vi "11-async.vi"() -> ()   [LabVIEW 2018, in "LV2Julia_examples.lvlib"]
uses:
  LV2Julia_examples.lvlib
  LV2Julia_core/VIs/Server or client state.ctl
  LV2Julia_core/VIs/detailed error info.ctl
  LV2Julia_core/VIs/StackFrame.ctl
  LV2Julia_core/VIs/Commands.ctl
  be4745b6-8471-45fc-b8a0-8968ce92ea4b.vi
  877f6708-f4bd-42a3-8abe-32eb8c2c970e.vi
  be4745b6-8471-45fc-b8a0-8968ce92ea4b.vi/01ce1741-ea78-47f8-98ed-e79163fb1a9b.vi
  877f6708-f4bd-42a3-8abe-32eb8c2c970e.vi/896d20f1-cb1d-4420-8f1f-f93355f5adea.vi
  be4745b6-8471-45fc-b8a0-8968ce92ea4b.vi/01ce1741-ea78-47f8-98ed-e79163fb1a9b.vi/cc3cf2af-bc3b-4fb6-855b-7562c4d0bfeb.vi
  be4745b6-8471-45fc-b8a0-8968ce92ea4b.vi/01ce1741-ea78-47f8-98ed-e79163fb1a9b.vi/c77cecd8-10de-4d46-bc1c-57302a887fda.vi
  be4745b6-8471-45fc-b8a0-8968ce92ea4b.vi/01ce1741-ea78-47f8-98ed-e79163fb1a9b.vi/2cafb1dd-d397-4b79-911a-06d102936120.vi
  877f6708-f4bd-42a3-8abe-32eb8c2c970e.vi/896d20f1-cb1d-4420-8f1f-f93355f5adea.vi/9892c125-836d-426b-b144-8af50d50507b.vi
  877f6708-f4bd-42a3-8abe-32eb8c2c970e.vi/896d20f1-cb1d-4420-8f1f-f93355f5adea.vi/80aac079-9052-42cf-b2c3-c29da6bba58d.vi
  877f6708-f4bd-42a3-8abe-32eb8c2c970e.vi/896d20f1-cb1d-4420-8f1f-f93355f5adea.vi/6d5e1d21-cb4d-4981-8d16-85d9352ac501.vi
  LV2Julia_core/VIs/jl-scripts path.vi
  LV2Julia_core/VIs/check ID validity.vi
  LV2Julia_core/VIs/bindata_descr to JSON.vi
  LV2Julia_core/VIs/check cluster field names.vi
  LV2Julia_core/VIs/concat JSON.vi
  LV2Julia_core/VIs/build request.vi
  LV2Julia_core/VIs/Parse server response.vi
  LV2Julia_core/VIs/log jl exceptions.vi
  LV2Julia_core/LV2Julia_core.lvlib
panel:
  out "done":bool
  out "ticket":i32
  in  "summands":cluster{"x":dbl, "y":dbl}={"x"=2.0, "y"=2.0}
  in  "next":bool
  out "x+y":dbl=nan
  out "detailed error info":T1
  out "current error":errorcluster
  out "final error":errorcluster
  out "short err code":u8
  in  "stop":bool
  out "ZMQ timeout":bool
  out "Julia script file path":path
  out "temporary script path":path
  out "Jl Server state":T3
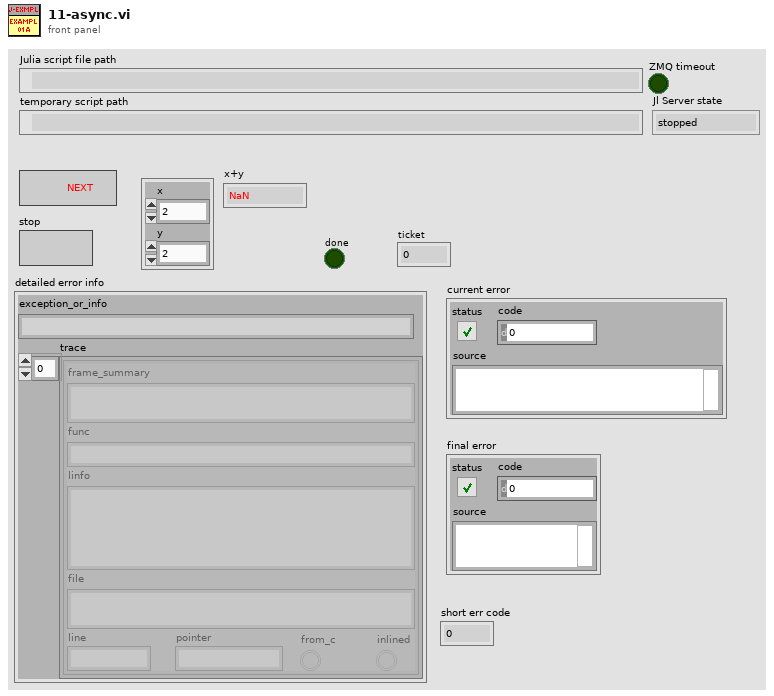
[diagram p1: front panel]
types:
  T1 = typedef "LV2Julia_core.lvlib/detailed error info.ctl" = cluster{"exception_or_info":string, "trace":T2[]}
  T2 = typedef "LV2Julia_core.lvlib/StackFrame.ctl" = cluster{"frame_summary":string, "func":string, "linfo":string, "file":string, "line":i32, "pointer":u64, "from_c":bool, "inlined":bool}
  T3 = typedef "LV2Julia_core.lvlib/Server or client state.ctl" = enum16{"stopped", "running", "unknown"}
  T4 = typedef "LV2Julia_core.lvlib/Commands.ctl" = enum16{"Start Jl-server & Init LV-client", "Send request & Get response ", "Stop Jl-server & Cleanup LV-client", "Cleanup LV-client", "Start Jl-server", "Stop Jl-server", "Init LV-Client", "Cleanup LV-Client", "(not allowed)", "Set LV Client state", "Set Jl Server state", "set ZMQ timeout", "read ZMQ timeout", "read-out state"}
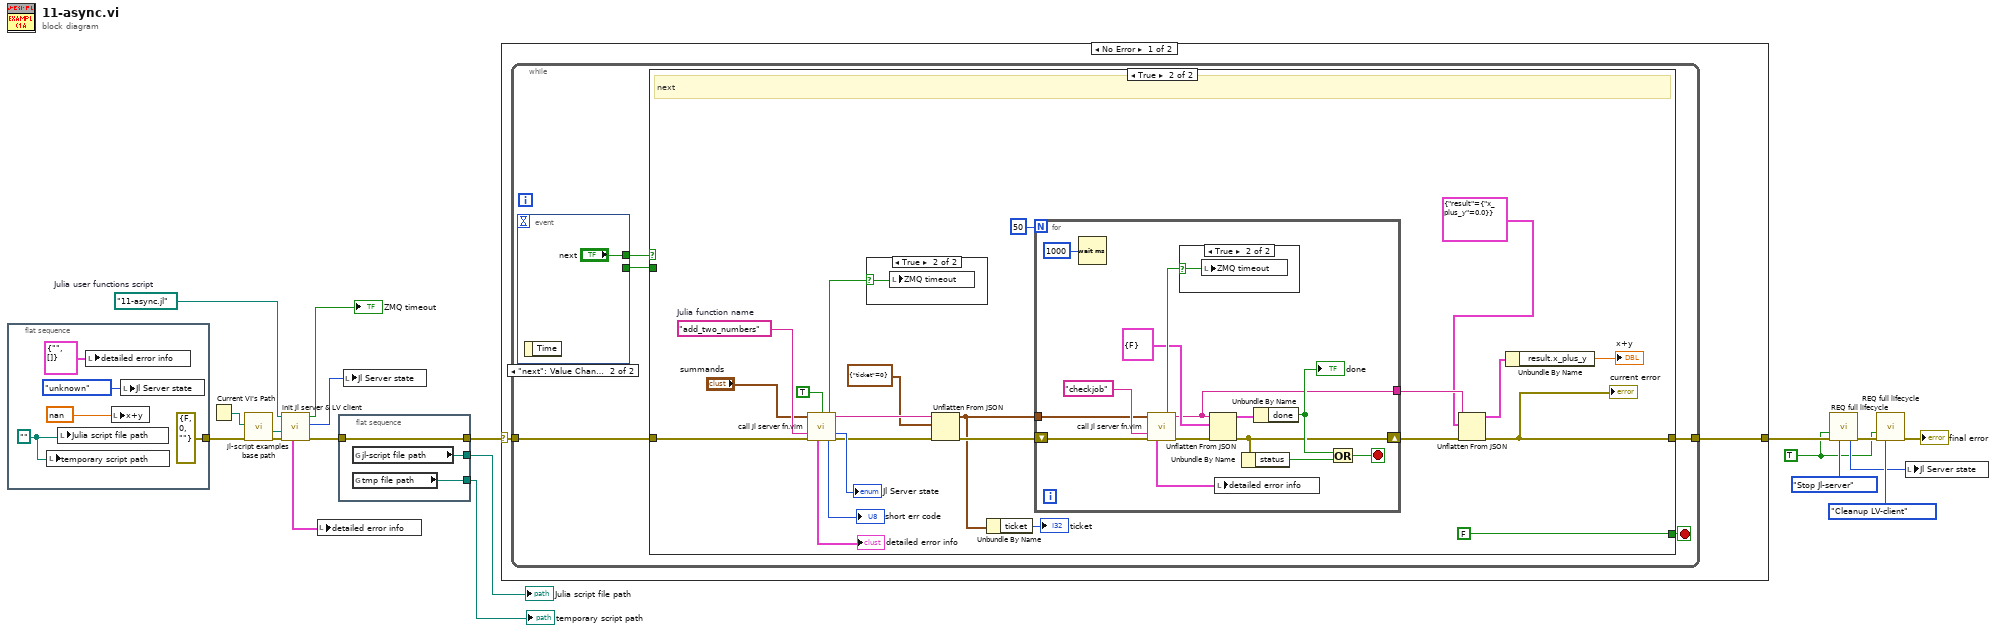
[diagram p0: block diagram]
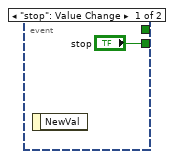
[diagram p2: hidden frame]
diagram:
  w10 = path "11-async.jl"  # Julia user functions script
  w9 = TRUE ("Force command")
  n1 = flat-sequence {
    tunnel: [errorcluster {"status"=FALSE, "code"=0, "source"=""} ("error in (no error)")] -> w5
    frame #0 {
      w20 = path ""
      n2 = local write "temporary script path"(w20) -> ()
      n3 = local write "Julia script file path"(w20) -> ()
      n4 = local write "detailed error info"(T1 {"exception_or_info"="", "trace"=[]} ("detailed error info")) -> ()
      n5 = local write "x+y"(nan ("Server response")) -> ()
      n6 = local write "Jl Server state"(Server_or_client_state."unknown" ("Jl Server state out")) -> ()
    }
  }
  n7 = Current VI's Path() -> (path=w2:path)
  n8 = call "jl-script examples base path.vi"("error in (no error)"=w5, "calling example VI path"=w2) -> ("error out"=w4:errorcluster, "jl-script-examples base path"=w3:path)  [unwired: 8 in]
  n9 = call "init Jl server & LV client.vi"("error in (no error)"=w4, "Base path (not a path)"=w3, "Julia user functions script"=w10) -> ("error out"=w7:errorcluster, "Jl Server state out"=w6:T3, "timeout?"=→"ZMQ timeout":bool, "detailed error info"=w1:T1)  [unwired: 3 in, 2 out]
  n10 = local write "detailed error info"(w1) -> ()
  n11 = flat-sequence {
    tunnel: [w27] -> w14
    tunnel: w7 -> [w27]
    tunnel: [w26] -> w12
    tunnel: [w25] -> w13
    frame #0 {
      n12 = global read "jl-scripts path.vi" "jl-script file path"() -> (w26:path)
      n13 = global read "jl-scripts path.vi" "tmp file path"() -> (w25:path)
    }
  }
  n14 = local write "Jl Server state"(w6) -> ()
  n15 = case shown="No Error" w14 {
    selector: w14 -> [w28 w77]
    tunnel: [w29 w77] -> w19
    frame No Error {
      n16 = while {
        tunnel: w28 -> [w33]
        tunnel: [w34] -> w29
        stop <- w31 stop-if-true
        n17 = event shown="[1] \"next\": Value Change" {
          selector: _ -> [_ _]
          dyn-events: _ -> [_ _]
          timeout: _ -> [_ _]
          tunnel: [_ "next"] -> w32
          tunnel: ["stop" _] -> w30
          event "stop": Value Change {
            n18 = event-data() -> ()  [unwired: 1 in, 1 out]
          }
          event "next": Value Change {
            n19 = event-data() -> ()  [unwired: 1 in, 1 out]
          }
        }
        n20 = case shown="True" w32 {
          tunnel: [w38 w50] -> w34
          tunnel: w33 -> [w38 w52]
          tunnel: [w37 FALSE ("stop this VI only")] -> w31
          tunnel: w30 -> [w37 _]
          frame False {
            # "stop"
          }
          frame True {
            w58 = "add_two_numbers"  # Julia function name
            # "next"
            n21 = call "call Jl server fn.vim"("Arguments 1"="summands", "async call (false)"=TRUE ("timeout?"), "fun2call"=w58, "error in (no error)"=w52) -> ("timeout?"=w55:bool, "JSON received"=w48:string, "Jl Server state out"=→"Jl Server state":T3, "detailed error info"=→"detailed error info":T1, "return code"=→"short err code":u8, "error out"=w47:errorcluster)  [unwired: 5 in, 1 out]
            n22 = case shown="True" w55 {
              selector: w55 -> [_ w76]
              frame False {
              }
              frame True {
                n23 = local write "ZMQ timeout"(w76) -> ()
              }
            }
            n24 = Unflatten From JSON(JSON string=w48, type and defaults=cluster{"ticket":i32} {"ticket"=0} ("parsed response"), error in (no error)=w47) -> (value=w44:cluster{"ticket":i32}, error out=w45:errorcluster)  [unwired: 4 in]
            n25 = Unbundle By Name(w44) -> ("ticket"=→"ticket":i32)
            n26 = for {
              N: 50 -> [_]
              tunnel: w44 -> [w72]
              tunnel: [w65] -> w42
              shift-right: [w64] -> w41
              shift-left: w45 -> [w73]
              stop <- w63 stop-if-true
              n27 = Wait (ms)(milliseconds to wait=u32 1000) -> ()  [unwired: 1 out]
              n28 = call "call Jl server fn.vim"("Arguments 1"=w72, "fun2call"="checkjob" ("Julia function name"), "error in (no error)"=w73) -> ("timeout?"=w71:bool, "JSON received"=w65:string, "detailed error info"=w61:T1, "error out"=w70:errorcluster)  [unwired: 6 in, 3 out]
              n29 = case shown="True" w71 {
                selector: w71 -> [_ w75]
                frame False {
                }
                frame True {
                  n30 = local write "ZMQ timeout"(w75) -> ()
                }
              }
              n31 = Unflatten From JSON(JSON string=w65, type and defaults=cluster{"done":bool} {"done"=FALSE}, error in (no error)=w70) -> (value=w67:cluster{"done":bool}, error out=w64:errorcluster)  [unwired: 4 in]
              n32 = local write "detailed error info"(w61) -> ()
              n33 = Unbundle By Name(w64) -> ("status"=w62:bool)
              n34 = Unbundle By Name(w67) -> ("done"=w66:bool)
              "done" <- w66
              n35 = Or(x=w66, y=w62) -> (x .or. y?=w63:bool)
            }
            n36 = Unflatten From JSON(JSON string=w42, type and defaults=cluster{"result":cluster{"x_plus_y":dbl}} {"result"={"x_plus_y"=0.0}}, error in (no error)=w41) -> (value=w51:cluster{"result":cluster{"x_plus_y":dbl}}, error out=w50:errorcluster)  [unwired: 4 in]
            "current error" <- w50
            n37 = Unbundle By Name(w51) -> ("result.x_plus_y"=→"x+y":dbl)
          }
        }
      }
    }
    frame Error {
    }
  }
  n38 = call "REQ full lifecycle.vi"("Force command"=w9, "error in"=w19, "command"=Commands."Stop Jl-server") -> ("Jl Server state out"=w11:T3, "error out"=w17:errorcluster)  [unwired: 6 in, 5 out]
  n39 = call "REQ full lifecycle.vi"("Force command"=w9, "error in"=w17, "command"=Commands."Cleanup LV-client") -> ("error out"=→"final error":errorcluster)  [unwired: 6 in, 6 out]
  n40 = local write "Jl Server state"(w11) -> ()
  "temporary script path" <- w13
  "Julia script file path" <- w12
